vi "ProdaNG.Global.vi"() -> ()   [LabVIEW 2016]
panel:
  in  "ErrorCode":i32=5500
  out "DbgLog":bool
  in  "DbgLogPath":path
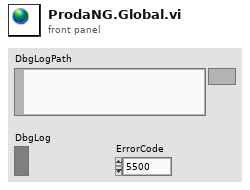
[diagram p1: front panel]
diagram:
